vi "Extract Single Tone Information 1 Chan.vi"(6 "advanced search":T4={"approx freq. (optional)"=-1.0, "search (+/- % of Fsampl.)"=5.0} {"search (+/- % of Fsampl.)" format="%0.2p"; "approx freq. (optional)" format="%0.2p"}, 8 "error in (no error)":errorcluster, 10 "export mode":T3(ring), 11 "time signal in":waveform(dbl)) -> (0 "error out":errorcluster, 1 "detected phase (deg)":dbl format="%.2p", 2 "detected amplitude":dbl format="%.2p", 3 "detected frequency":dbl format="%.2p", 4 "measurement info":T2={"uncertainty"=0.0, "Warning"=FALSE, "comments"="reserved for future use"} {"uncertainty" format="%0.2p"}, 5 "exported signals":T1 {"exported spectrum (dB)"."dB Spectrum (Hann)" format="%.2p"; "exported spectrum (dB)"."df" format="%.2p"; "exported spectrum (dB)"."f0" format="%.2p"})   [LabVIEW 2020, in "NI_MAPro.lvlib"]
doc: "Takes a signal in, finds the single tone with the highest amplitude or searches a specified frequency range, and returns the single tone frequency, amplitude, and phase. The input signal can be real or complex and single-channel or multichannel. Wire data to the <B>time signal in</B> input to determine the polymorphic instance to use or manually select the instance."
uses:
  NI_MAPro.lvlib
  NI_MABase.lvlib
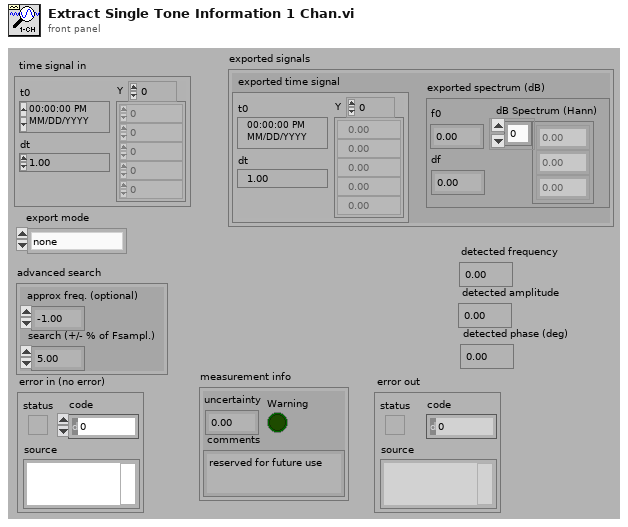
[diagram p1: front panel]
types:
  T1 = cluster{"exported time signal":waveform(dbl), "exported spectrum (dB)":cluster{"f0":dbl, "df":dbl, "dB Spectrum (Hann)":dbl[]}}
  T2 = cluster{"uncertainty":dbl, "Warning":bool, "comments":string}
  T3 = enum32{"none", "input signal", "detected signal", "residual signal"}
  T4 = cluster{"approx freq. (optional)":dbl, "search (+/- % of Fsampl.)":dbl}
  T5 = cluster{"f0":dbl, "df":dbl, "dB Spectrum (Hann)":dbl[]}
  T6 = cluster{"time signal in":waveform(dbl), "exported spectrum (dB)":cluster{"f0":dbl, "df":dbl, "dB Spectrum (Hann)":dbl[]}}
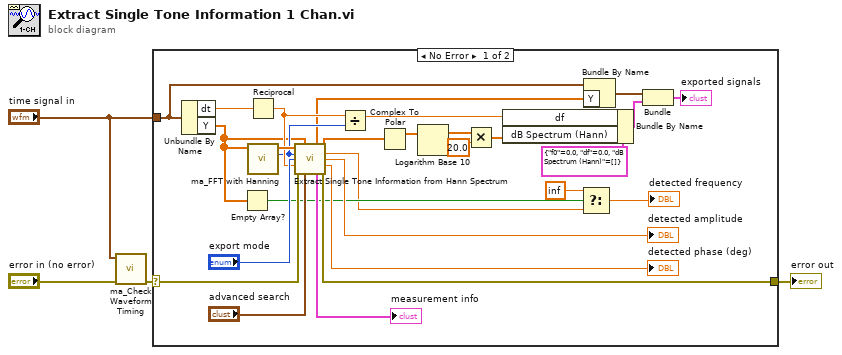
[diagram p0: block diagram]
diagram:
  n1 = call "ma_Check Waveform Timing.vi"("error in (no error)"="error in (no error)", "signal in"="time signal in") -> ("error out"=w2:errorcluster)  [unwired: 1 in, 8 out]
  n2 = case shown="No Error" w2 {
    selector: w2 -> [w11 w33]
    tunnel: "time signal in" -> [w15 _]
    tunnel: [w10 w33] -> w4
    frame No Error {
      n3 = Unbundle By Name(w15) -> ("dt"=w16:dbl, "Y"=w9:dbl[])
      n4 = Empty Array?(array=w9) -> (empty?=w8:bool)
      n5 = Reciprocal(x=w16) -> (1/x=w19:dbl)
      n6 = call "ma_FFT with Hanning.vi"("time signal data"=w9) -> ("FFT size"=w18:i32, "complex Hann spectrum"=w28:cdb[])  [unwired: 2 in, 7 out]
      n7 = call "Extract Single Tone Information from Hann Spectrum.vi"("complex spectrum in"=w28, "time signal in"=w9, "FFT size"=w18, "export mode"="export mode", "sampling frequency"=w19, "error in"=w11, "advanced search"="advanced search") -> ("time signal out"=w14:dbl[], "complex spectrum out"=w20:cdb[], "detected frequency"=w6:dbl, "detected amplitude"=→"detected amplitude":dbl, "detected phase (deg)"=→"detected phase (deg)":dbl, "measurement info"=→"measurement info":T2, "error out"=w10:errorcluster)  [unwired: 2 out]
      n8 = Divide(x=w19, y=w18) -> (x/y=w17:dbl)
      n9 = Complex To Polar(r * e^(i*theta)=w20) -> (r=w24:dbl[])  [unwired: 1 out]
      n10 = Logarithm Base 10(1:w24) -> (0:w23:dbl[])
      n11 = Multiply(x=w23, y=20.0) -> (x*y=w21:dbl[])
      n12 = Bundle By Name(cluster=T5 {"f0"=0.0, "df"=0.0, "dB Spectrum (Hann)"=[]} ("exported spectrum (dB)"), "df"=w17, "dB Spectrum (Hann)"=w21) -> (w26:T5)
      n13 = Select(t=inf, s=w8, f=w6) -> (s? t:f=→"detected frequency":dbl)
      n14 = Bundle By Name(cluster=w15, "Y"=w14) -> (w13:waveform(dbl))
      n15 = Bundle("time signal in"=w13, "exported spectrum (dB)"=w26) -> (→"exported signals":T6)  [unwired: 1 out]
    }
    frame Error {
    }
  }
  "error out" <- w4
